vi "GetSelectedSigValInDraw.vi"(9 "值表数组":string[][](array[string]), 10 "已选信号列表":string[][](array[string])) -> (1 "已选信号值定义数组":string[][](array[string]))   [LabVIEW 2015]
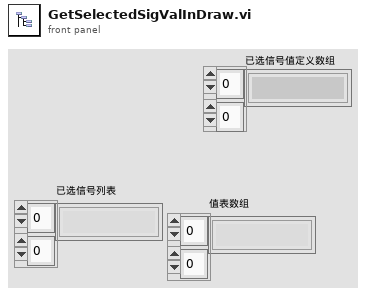
[diagram p1: front panel]
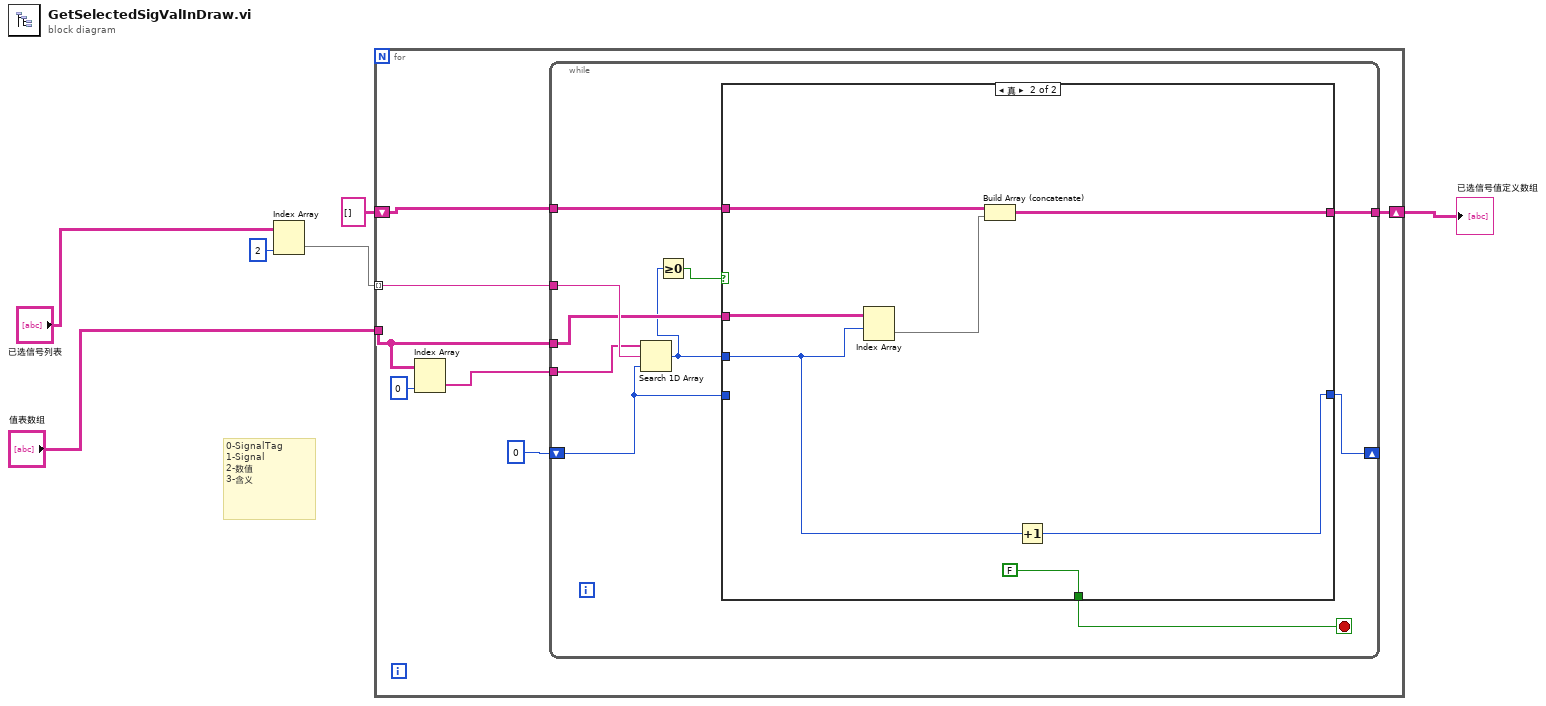
[diagram p0: block diagram]
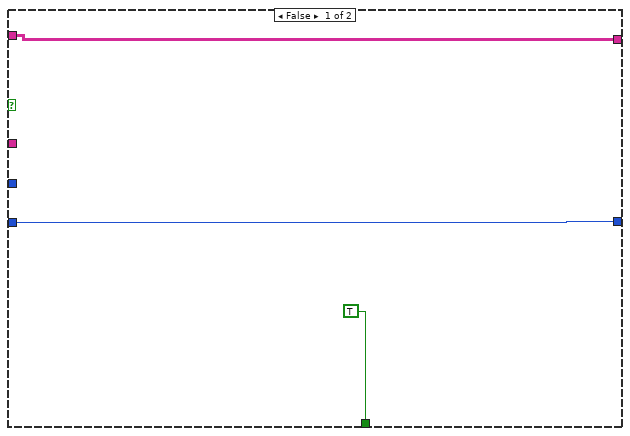
[diagram p2: hidden frame]
diagram:
  # "0-SignalTag\n1-Signal\n2-数值\n3-含义"
  n1 = Index Array(array="已选信号列表", index (col)=2 ("禁用的索引 (列)")) -> (element=w4:string[])  [unwired: 1 in]
  n2 = for {
    tunnel: w4 -> [w13] mode=indexing
    tunnel: "值表数组" -> [w9]
    shift-right: [w8] -> w1
    shift-left: string[][] [] -> [w7]
    n3 = Index Array(array=w9, index (col)=0 ("禁用的索引 (列)")) -> (element=w10:string[])  [unwired: 1 in]
    n4 = while {
      tunnel: w13 -> [w23]
      tunnel: w9 -> [w22]
      shift-right: [w19] -> _
      shift-left: 0 -> [w18]
      tunnel: w10 -> [w16]
      tunnel: [w15] -> w8
      tunnel: w7 -> [w14]
      stop <- w17 stop-if-true
      n5 = Search 1D Array(1D array=w16, element=w23, start index (0)=w18) -> (index of element=w21:i32)
      n6 = Greater Or Equal To 0?(x=w21) -> (x >= 0?=w20:bool)
      n7 = case shown="真" w20 {
        tunnel: w22 -> [_ w31]
        tunnel: w21 -> [_ w30]
        tunnel: [w26 w33] -> w19
        tunnel: w18 -> [w26 _]
        tunnel: [TRUE FALSE] -> w17
        tunnel: [w24 w28] -> w15
        tunnel: w14 -> [w24 w27]
        frame False {
        }
        frame True {
          n8 = Index Array(array=w31, index (row)=w30) -> (element=w29:string[])  [unwired: 1 in]
          n9 = Build Array (concatenate)(w27, w29) -> (w28:string[][])
          n10 = Increment(x=w30) -> (x+1=w33:i32)
        }
      }
    }
  }
  "已选信号值定义数组" <- w1
